vi "AD9959controlMR1_B2.vi"(9 "Enable Master Stepper":bool, 10 "Array":T2(array[cluster]) {"Sweep Parameters"."Rising Step Interval (ms)" min=0.0 max=2.55 step=0.01 format="%.2f"; "Sweep Parameters"."Stop Frequency (MHz)" min=0.0 max=400.0 step=1.0 format="%.6f"; "Sweep Parameters"."Start Frequency (MHz)" min=0.0 max=400.0 step=1.0 format="%.6f"; "Sweep Parameters"."Falling Step Interval (ms)" min=0.0 max=2.55 step=0.01 format="%.2f"; "Sweep Parameters"."Falling Step Size (MHz)" min=0.0 max=400.0 step=0.1 format="%.6f"; "Sweep Parameters"."Rising Step Size (MHz)" min=0.0 max=400.0 step=0.1 format="%.6f"; "ASF" min=0.0 max=1.0 step=0.001 format="%.3f"; "Channel Frequency (MHz)" min=0.0 max=400.0 step=1.0 format="%.6f"}, 11 "VISA Reference":refnum<visa-resource-name>="AD2") -> (2 "Duration array":T1(array[cluster]))   [LabVIEW 2016]
uses:
  <userlib>/configTool/configTool.llb/initConfigGlobal.vi
  <userlib>/configTool/configTool.llb/addProperty(DBL).vi
  <userlib>/configTool/configTool.llb/addProperty(BOOL).vi
  <userlib>/configTool/configTool.llb/saveConfigFile - Text.vi
  <userlib>/configTool/configTool.llb/closeConfig.vi
panel:
  out "Actual Channel Frequencies (MHz)":dbl[](array[numeric]) format="%#_10g"
  out "error out 2":errorcluster
  in  "config file path":path
  in  "Save Config File":bool=TRUE
  in  "Load Config File?":bool=TRUE
  out "System Clock (MHz)":u32
  in  "Multiplier":u32=5
  in  "Reference Clock (MHz)":u32=20
  # "AD2"
  # "AOM3    IntraAction 110 MHz\nRepump"
  # "AOM3    IntraAction 110MHz    \nWrite"
  # "AOM2   IntraAction 110 MHz\nRead"
  # "AOM7 Isomet 80MHz\nSPAD Gate"
  # "max 0.140"
  # "max 0.15"
  # "max 0.175"
  # "max 0.090/ 0.25 for LW"
  # "Channel 1"
  # "Channel 2"
  # "Channel 3"
  # "Channel 0"
  # "I/O"
  # "Clock"
  # "Profile Pins"
  # "P0 is uncut\nP1 is uncut\nP2 is uncut\nP3 is uncut"
  # "Power Down"
  # "Notes:\nMinimum Frequency Step is 0.0931 Hz.\nMinimum ASF Step is 0.001"
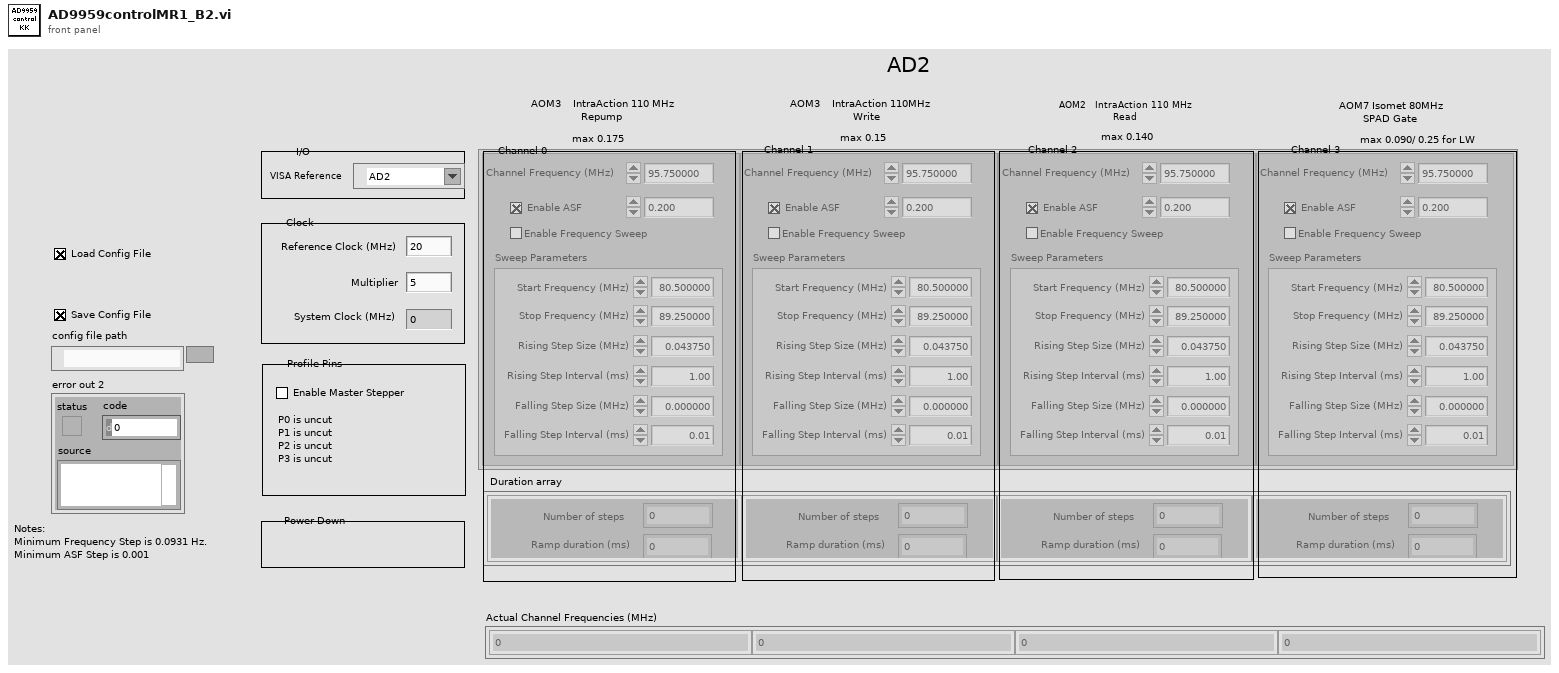
[diagram p1: front panel]
types:
  T1 = cluster{"Number of steps":dbl, "Ramp duration (ms)":dbl}[]
  T2 = cluster{"Enable ASF?":bool, "Channel Frequency (MHz)":dbl, "ASF":dbl, "Enable Frequency Sweep":bool, "Sweep Parameters":cluster{"Start Frequency (MHz)":dbl, "Stop Frequency (MHz)":dbl, "Rising Step Size (MHz)":dbl, "Falling Step Size (MHz)":dbl, "Falling Step Interval (ms)":dbl, "Rising Step Interval (ms)":dbl}}[]
  T3 = cluster{"Start Frequency (MHz)":dbl, "Stop Frequency (MHz)":dbl, "Rising Step Size (MHz)":dbl, "Falling Step Size (MHz)":dbl, "Falling Step Interval (ms)":dbl, "Rising Step Interval (ms)":dbl}[]
  T4 = cluster{"# of steps":dbl, "Ramp duration (ms)":dbl}[]
  T5 = cluster{"# of steps":dbl, "Ramp duration (ms)":dbl}
  T6 = cluster{"Start Frequency (MHz)":dbl, "Stop Frequency (MHz)":dbl, "Rising Step Size (MHz)":dbl, "Falling Step Size (MHz)":dbl, "Falling Step Interval (ms)":dbl, "Rising Step Interval (ms)":dbl}
  T7 = typedef "configRef.ctl" = refnum<vi>
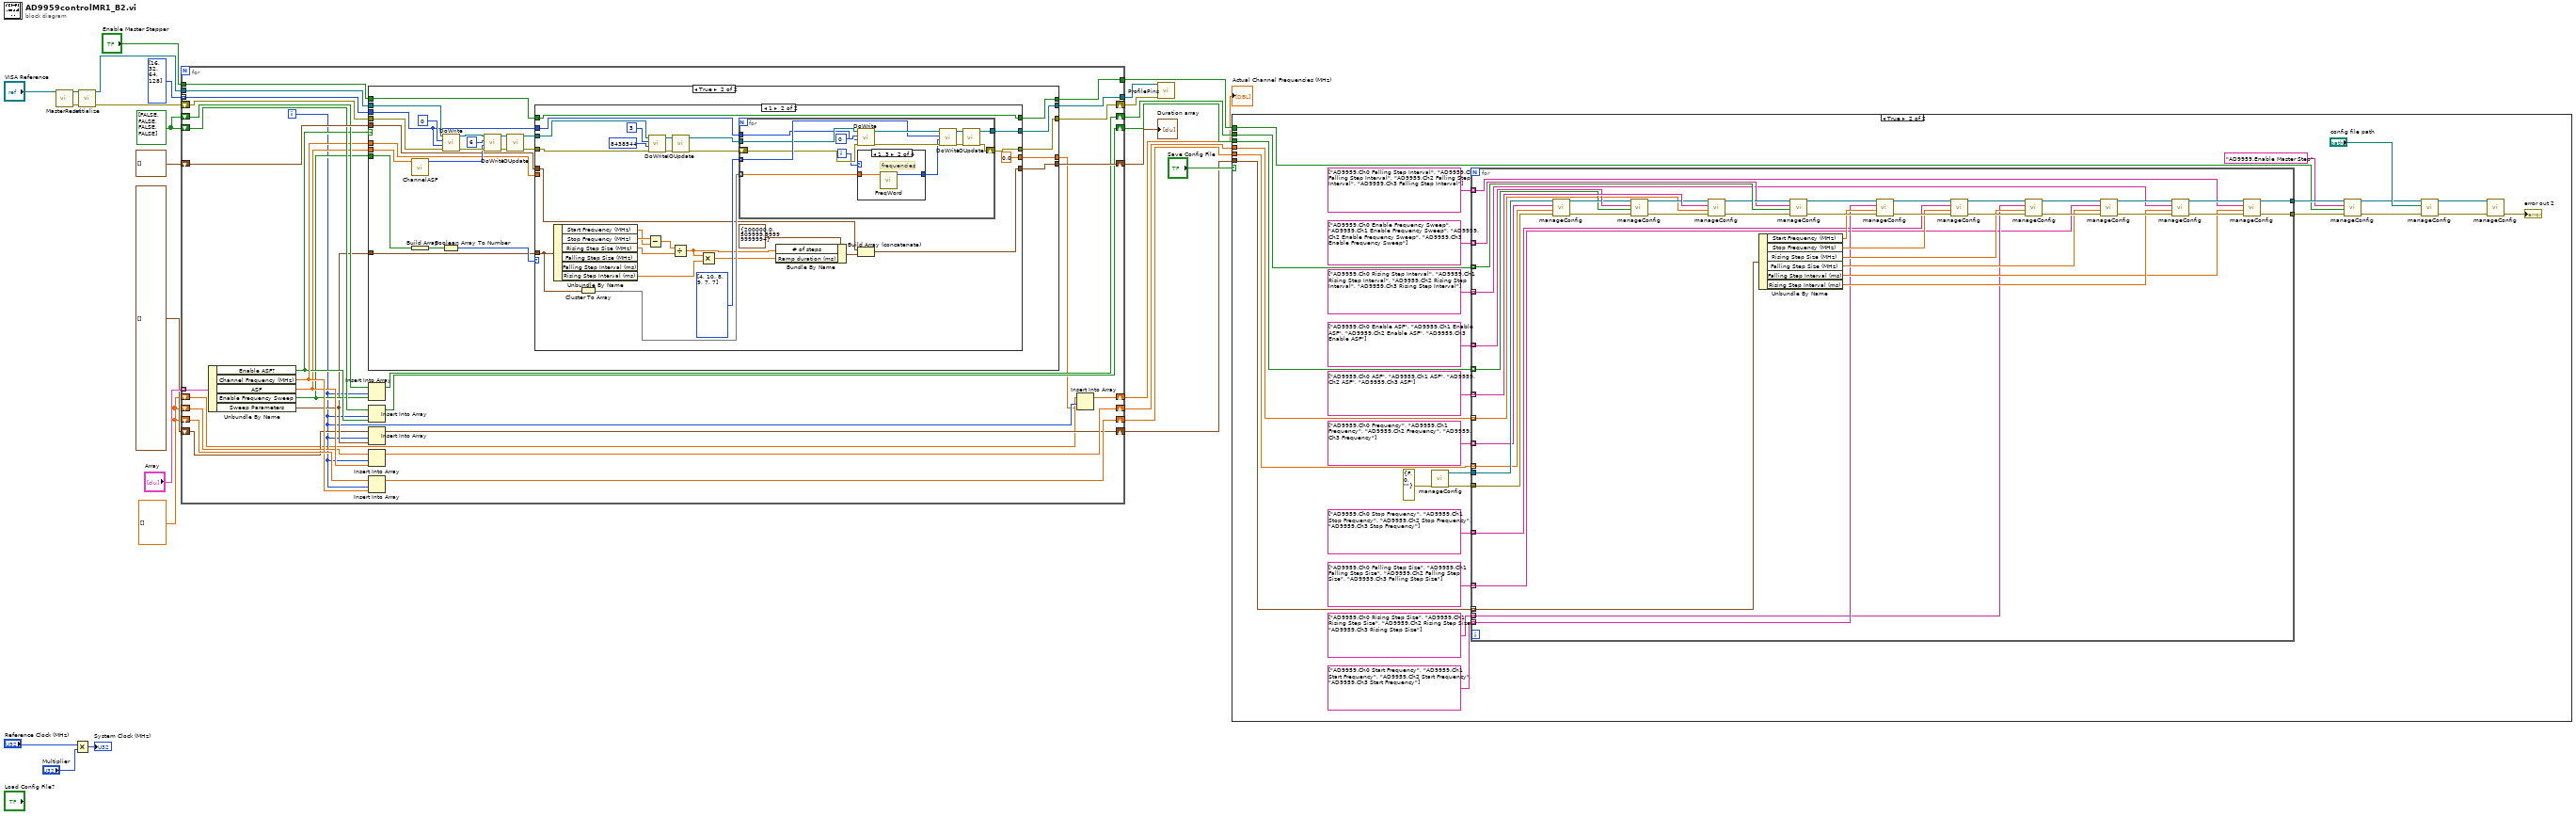
[diagram p0: block diagram]
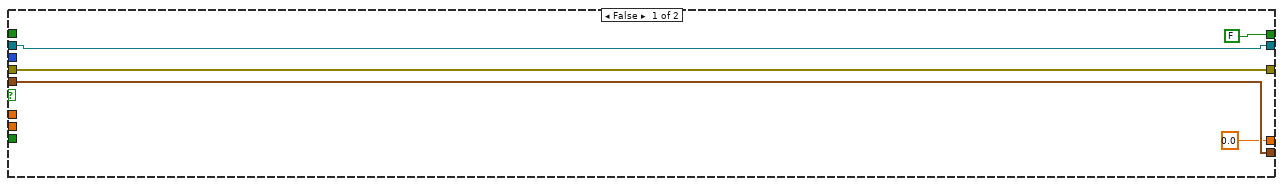
[diagram p3: hidden frame]
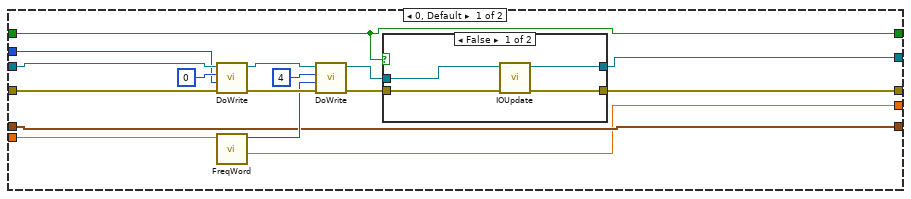
[diagram p4: hidden frame]
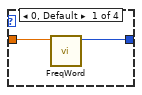
[diagram p6: hidden frame]
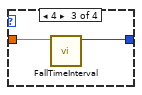
[diagram p7: hidden frame]
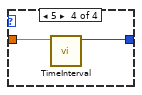
[diagram p8: hidden frame]
diagram:
  w2 = dbl[] [] ("array")
  w12 = bool[] [FALSE, FALSE, FALSE, FALSE] ("element")
  n1 = call "MasterReset.vi"("VISA Reference"="VISA Reference") -> ("error out"=w21:errorcluster, "dup VISA resource name"=w22:refnum<visa-resource-name>)  [unwired: 9 in]
  n2 = Multiply(x="Reference Clock (MHz)", y="Multiplier") -> (x*y=→"System Clock (MHz)":u32)
  n3 = call "Initialize.vi"("error in (no error)"=w21, "VISA Reference"=w22) -> ("error out"=w18:errorcluster, "dup VISA resource name"=w4:refnum<visa-resource-name>)  [unwired: 8 in]
  n4 = for {
    tunnel: "Array" -> [w55] mode=indexing
    tunnel: [w54] -> w3
    tunnel: w4 -> [w53]
    tunnel: u32[] [16, 32, 64, 128] ("Value 3") -> [w51] mode=indexing
    shift-right: [w50] -> w15
    shift-left: T4 [] -> [w49]
    shift-right: [w48] -> w19
    shift-left: w18 -> [w52]
    shift-right: [w46] -> w13
    shift-left: w12 -> [w47]
    shift-right: [w44] -> w11
    shift-left: w12 -> [w45]
    shift-right: [w41] -> w10
    shift-left: w2 -> [w43]
    shift-right: [w37] -> w8
    shift-left: w2 -> [w38]
    shift-right: [w33] -> w7
    shift-left: T3 [] ("array") -> [w34]
    tunnel: [w32] -> w6
    tunnel: "Enable Master Stepper" -> [w31]
    shift-right: [w28] -> w1
    shift-left: w2 -> [w29]
    i -> [w30]
    n5 = Unbundle By Name(w55) -> ("Enable ASF?"=w40:bool, "Channel Frequency (MHz)"=w42:dbl, "ASF"=w39:dbl, "Enable Frequency Sweep"=w36:bool, "Sweep Parameters"=w35:T6)
    n6 = case shown="True" w40 {
      tunnel: w53 -> [w60 w82]
      tunnel: w52 -> [w59 w83]
      tunnel: [w60 w74] -> w54
      tunnel: [w59 w73] -> w48
      tunnel: w39 -> [_ w72]
      tunnel: w36 -> [_ w67]
      tunnel: w42 -> [_ w71]
      tunnel: w35 -> [_ w62]
      tunnel: w51 -> [_ w70]
      tunnel: [w58 w66] -> w50
      tunnel: w49 -> [w58 w65]
      tunnel: [FALSE ("Enable Master Stepper") w64] -> w32
      tunnel: w31 -> [_ w63]
      tunnel: [0.0 ("Actual Frequency (MHz)") w61] -> w27
      frame False {
      }
      frame True {
        n7 = call "ChannelASF.vi"("ASF"=w72) -> ("ASF in hex"=w76:u32)  [unwired: 10 in]
        n8 = Build Array(w67) -> (w68:bool[])
        n9 = Boolean Array To Number(Boolean array=w68) -> (number=w69:u32)
        n10 = call "DoWrite.vi"("error in (no error)"=w83, "Value"=w70, "Register Address"=0 ("Value 3"), "VISA Reference"=w82) -> ("error out"=w79:errorcluster, "dup VISA resource name"=w81:refnum<visa-resource-name>)  [unwired: 6 in]
        n11 = call "DoWrite.vi"("error in (no error)"=w79, "Value"=w76, "Register Address"=u32 6 ("Register Address 4"), "VISA Reference"=w81) -> ("error out"=w77:errorcluster, "dup VISA resource name"=w80:refnum<visa-resource-name>)  [unwired: 6 in]
        n12 = call "IOUpdate.vi"("error in (no error)"=w77, "VISA Reference"=w80) -> ("error out"=w84:errorcluster, "dup VISA resource name"=w85:refnum<visa-resource-name>)  [unwired: 8 in]
        n13 = case shown="1" w69 {
          tunnel: w84 -> [w94 w131]
          tunnel: w85 -> [w101 w132]
          tunnel: [w92 w124] -> w74
          tunnel: [w91 w123] -> w73
          tunnel: w71 -> [w90 _]
          tunnel: w62 -> [_ w121]
          tunnel: w70 -> [w89 w122]
          tunnel: [w88 w110] -> w66
          tunnel: w65 -> [w88 w113]
          tunnel: [w87 w109] -> w64
          tunnel: w63 -> [w87 w109]
          tunnel: [w86 0.0 ("Actual Frequency (MHz)")] -> w61
          frame 0, Default {
            n14 = call "DoWrite.vi"("error in (no error)"=w94, "Value"=w89, "Register Address"=0 ("Value 3"), "VISA Reference"=w101) -> ("error out"=w100:errorcluster, "dup VISA resource name"=w99:refnum<visa-resource-name>)  [unwired: 6 in]
            n15 = call "FreqWord.vi"("Channel Frequency (MHz)"=w90) -> ("Actual Frequency (MHz)"=w86:dbl, "Frequency Tuning Word"=w95:u32)  [unwired: 9 in]
            n16 = call "DoWrite.vi"("error in (no error)"=w100, "Value"=w95, "Register Address"=u32 4 ("Register Address 2"), "VISA Reference"=w99) -> ("error out"=w97:errorcluster, "dup VISA resource name"=w98:refnum<visa-resource-name>)  [unwired: 6 in]
            n17 = case shown="False" w87 {
              tunnel: w98 -> [w105 w107]
              tunnel: w97 -> [w104 w106]
              tunnel: [w103 w107] -> w92
              tunnel: [w102 w106] -> w91
              frame False {
                n18 = call "IOUpdate.vi"("error in (no error)"=w104, "VISA Reference"=w105) -> ("error out"=w102:errorcluster, "dup VISA resource name"=w103:refnum<visa-resource-name>)  [unwired: 8 in]
              }
              frame True {
              }
            }
          }
          frame 1 {
            n19 = Unbundle By Name(w121) -> ("Start Frequency (MHz)"=w119:dbl, "Stop Frequency (MHz)"=w120:dbl, "Rising Step Size (MHz)"=w118:dbl, "Rising Step Interval (ms)"=w117:dbl)  [unwired: 2 out]
            n20 = Cluster To Array(cluster=w121) -> (array=w127:dbl[])
            n21 = Subtract(x=w120, y=w119) -> (x-y=w116:dbl)
            n22 = call "DoWrite.vi"("error in (no error)"=w131, "Value"=8438544 ("Value 3"), "Register Address"=3 ("Value 3"), "VISA Reference"=w132) -> ("error out"=w134:errorcluster, "dup VISA resource name"=w133:refnum<visa-resource-name>)  [unwired: 6 in]
            n23 = Divide(x=w116, y=w118) -> (x/y=w112:dbl)
            n24 = call "IOUpdate.vi"("error in (no error)"=w134, "VISA Reference"=w133) -> ("error out"=w126:errorcluster, "dup VISA resource name"=w125:refnum<visa-resource-name>)  [unwired: 8 in]
            n25 = Multiply(x=w112, y=w117) -> (x*y=w111:dbl)
            n26 = for {
              tunnel: i32[] [4, 10, 8, 9, 7, 7] -> [w144] mode=indexing
              shift-right: [w143] -> w123
              shift-left: w126 -> [w142]
              tunnel: w125 -> [w141]
              tunnel: [w136] -> w124
              tunnel: w127 -> [w138] mode=indexing
              tunnel: w122 -> [w135]
              i -> [w139]
              n27 = call "DoWrite.vi"("error in (no error)"=w142, "Value"=w135, "Register Address"=0 ("Value 3"), "VISA Reference"=w141) -> ("error out"=w145:errorcluster, "dup VISA resource name"=w146:refnum<visa-resource-name>)  [unwired: 6 in]
              n28 = case shown="1..3" w139 {
                tunnel: w138 -> [w150 w152 w154 w156]
                tunnel: [w149 w151 w153 w155] -> w137
                frame 0, Default {
                  n29 = call "FreqWord.vi"("Channel Frequency (MHz)"=w150) -> ("Frequency Tuning Word"=w149:u32)  [unwired: 9 in, 1 out]
                }
                frame 1..3 {
                  # "frequencies"
                  n30 = call "FreqWord.vi"("Channel Frequency (MHz)"=w152) -> ("Frequency Tuning Word"=w151:u32)  [unwired: 9 in, 1 out]
                }
                frame 4 {
                  n31 = call "FallTimeInterval.vi"("Fall Time Interval"=w154) -> ("Time interval in Hex"=w153:u32)  [unwired: 10 in]
                }
                frame 5 {
                  n32 = call "TimeInterval.vi"("Time Interval"=w156) -> ("Time interval in Hex"=w155:u32)  [unwired: 10 in]
                }
              }
              n33 = call "DoWrite.vi"("error in (no error)"=w145, "Value"=w137, "Register Address"=w144, "VISA Reference"=w146) -> ("error out"=w147:errorcluster, "dup VISA resource name"=w148:refnum<visa-resource-name>)  [unwired: 6 in]
              n34 = call "IOUpdate.vi"("error in (no error)"=w147, "VISA Reference"=w148) -> ("error out"=w143:errorcluster, "dup VISA resource name"=w136:refnum<visa-resource-name>)  [unwired: 8 in]
            }
            n35 = Bundle By Name(cluster=T5 {"# of steps"=200000.0, "Ramp duration (ms)"=509999.99999999994} ("Duration Cluster"), "# of steps"=w112, "Ramp duration (ms)"=w111) -> (w115:T5)
            n36 = Build Array (concatenate)(w113, w115) -> (w110:T4)
          }
        }
      }
    }
    n37 = Insert Into Array(array=w45, index=w30, new element=w36) -> (w44:bool[])
    n38 = Insert Into Array(array=w47, index=w30, new element=w40) -> (w46:bool[])
    n39 = Insert Into Array(array=w34, index=w30, new element=w35) -> (w33:T3)
    n40 = Insert Into Array(array=w38, index=w30, new element=w39) -> (w37:dbl[])
    n41 = Insert Into Array(array=w43, index=w30, new element=w42) -> (w41:dbl[])
    n42 = Insert Into Array(array=w29, index=w30, new element=w27) -> (w28:dbl[])
  }
  "Duration array" <- w15
  "Actual Channel Frequencies (MHz)" <- w1
  n43 = call "ProfilePins.vi"("error in (no error)"=w19, "VISA Reference"=w3) -> ()  [unwired: 8 in, 2 out]
  n44 = case shown="True" "Save Config File" {
    tunnel: w13 -> [_ w177]
    tunnel: w11 -> [_ w175]
    tunnel: w10 -> [_ w172]
    tunnel: w8 -> [_ w171]
    tunnel: w7 -> [_ w169]
    tunnel: w6 -> [_ w157]
    frame False {
    }
    frame True {
      n45 = call-poly <userlib>:"manageConfig.vi"("error in (no error)"=errorcluster {"status"=FALSE, "code"=0, "source"=""}) -> ("error out"=w174:errorcluster, "config ref out"=w179:T7)  [unwired: 9 in]
      n46 = for {
        tunnel: w179 -> [w222]
        tunnel: [w186] -> w162
        tunnel: string[] ["AD9959.Ch0 ASF", "AD9959.Ch1 ASF", "AD9959.Ch2 ASF", "AD9959.Ch3 ASF"] ("property path") -> [w227] mode=indexing
        tunnel: w177 -> [w217] mode=indexing
        tunnel: [w185] -> w161
        tunnel: string[] ["AD9959.Ch0 Enable ASF", "AD9959.Ch1 Enable ASF", "AD9959.Ch2 Enable ASF", "AD9959.Ch3 Enable ASF"] ("property path") -> [w225] mode=indexing
        tunnel: w175 -> [w214] mode=indexing
        tunnel: w174 -> [w220]
        tunnel: string[] ["AD9959.Ch0 Frequency", "AD9959.Ch1 Frequency", "AD9959.Ch2 Frequency", "AD9959.Ch3 Frequency"] ("property path") -> [w219] mode=indexing
        tunnel: w172 -> [w218] mode=indexing
        tunnel: w171 -> [w216] mode=indexing
        tunnel: string[] ["AD9959.Ch0 Enable Frequency Sweep", "AD9959.Ch1 Enable Frequency Sweep", "AD9959.Ch2 Enable Frequency Sweep", "AD9959.Ch3 Enable Frequency Sweep"] ("property path") -> [w212] mode=indexing
        tunnel: w169 -> [w211] mode=indexing
        tunnel: string[] ["AD9959.Ch0 Start Frequency", "AD9959.Ch1 Start Frequency", "AD9959.Ch2 Start Frequency", "AD9959.Ch3 Start Frequency"] ("property path") -> [w192] mode=indexing
        tunnel: string[] ["AD9959.Ch0 Stop Frequency", "AD9959.Ch1 Stop Frequency", "AD9959.Ch2 Stop Frequency", "AD9959.Ch3 Stop Frequency"] ("property path") -> [w191] mode=indexing
        tunnel: string[] ["AD9959.Ch0 Rising Step Size", "AD9959.Ch1 Rising Step Size", "AD9959.Ch2 Rising Step Size", "AD9959.Ch3 Rising Step Size"] ("property path") -> [w190] mode=indexing
        tunnel: string[] ["AD9959.Ch0 Falling Step Size", "AD9959.Ch1 Falling Step Size", "AD9959.Ch2 Falling Step Size", "AD9959.Ch3 Falling Step Size"] ("property path") -> [w189] mode=indexing
        tunnel: string[] ["AD9959.Ch0 Rising Step Interval", "AD9959.Ch1 Rising Step Interval", "AD9959.Ch2 Rising Step Interval", "AD9959.Ch3 Rising Step Interval"] ("property path") -> [w188] mode=indexing
        tunnel: string[] ["AD9959.Ch0 Falling Step Interval", "AD9959.Ch1 Falling Step Interval", "AD9959.Ch2 Falling Step Interval", "AD9959.Ch3 Falling Step Interval"] ("property path") -> [w187] mode=indexing
        n47 = call-poly <userlib>:"manageConfig.vi"("error in (no error)"=w220, "value"=w218, "property path"=w219, "config ref"=w222) -> ("error out"=w221:errorcluster, "config ref out"=w223:T7)  [unwired: 6 in]
        n48 = call-poly <userlib>:"manageConfig.vi"("error in (no error)"=w221, "value"=w217, "property path"=w225, "config ref"=w223) -> ("error out"=w224:errorcluster, "config ref out"=w226:T7)  [unwired: 6 in]
        n49 = call-poly <userlib>:"manageConfig.vi"("error in (no error)"=w224, "value"=w216, "property path"=w227, "config ref"=w226) -> ("error out"=w215:errorcluster, "config ref out"=w213:T7)  [unwired: 6 in]
        n50 = Unbundle By Name(w211) -> ("Start Frequency (MHz)"=w198:dbl, "Stop Frequency (MHz)"=w197:dbl, "Rising Step Size (MHz)"=w196:dbl, "Falling Step Size (MHz)"=w195:dbl, "Falling Step Interval (ms)"=w193:dbl, "Rising Step Interval (ms)"=w194:dbl)
        n51 = call-poly <userlib>:"manageConfig.vi"("error in (no error)"=w215, "value"=w214, "property path"=w212, "config ref"=w213) -> ("error out"=w199:errorcluster, "config ref out"=w200:T7)  [unwired: 6 in]
        n52 = call-poly <userlib>:"manageConfig.vi"("error in (no error)"=w199, "value"=w198, "property path"=w192, "config ref"=w200) -> ("error out"=w205:errorcluster, "config ref out"=w210:T7)  [unwired: 6 in]
        n53 = call-poly <userlib>:"manageConfig.vi"("error in (no error)"=w205, "value"=w197, "property path"=w191, "config ref"=w210) -> ("error out"=w204:errorcluster, "config ref out"=w209:T7)  [unwired: 6 in]
        n54 = call-poly <userlib>:"manageConfig.vi"("error in (no error)"=w204, "value"=w196, "property path"=w190, "config ref"=w209) -> ("error out"=w203:errorcluster, "config ref out"=w208:T7)  [unwired: 6 in]
        n55 = call-poly <userlib>:"manageConfig.vi"("error in (no error)"=w203, "value"=w195, "property path"=w189, "config ref"=w208) -> ("error out"=w202:errorcluster, "config ref out"=w207:T7)  [unwired: 6 in]
        n56 = call-poly <userlib>:"manageConfig.vi"("error in (no error)"=w202, "value"=w194, "property path"=w188, "config ref"=w207) -> ("error out"=w201:errorcluster, "config ref out"=w206:T7)  [unwired: 6 in]
        n57 = call-poly <userlib>:"manageConfig.vi"("error in (no error)"=w201, "value"=w193, "property path"=w187, "config ref"=w206) -> ("error out"=w185:errorcluster, "config ref out"=w186:T7)  [unwired: 6 in]
      }
      n58 = call-poly <userlib>:"manageConfig.vi"("error in (no error)"=w161, "value"=w157, "property path"="AD9959.Enable Master Step", "config ref"=w162) -> ("error out"=w160:errorcluster, "config ref out"=w159:T7)  [unwired: 6 in]
      n59 = call-poly <userlib>:"manageConfig.vi"("error in"=w160, "config file path"="config file path", "config ref"=w159) -> ("error out"=w184:errorcluster, "config ref out"=w183:T7)  [unwired: 6 in, 1 out]
      n60 = call-poly <userlib>:"manageConfig.vi"("error in (no error)"=w184, "config ref"=w183) -> ("error out"=→"error out 2":errorcluster)  [unwired: 9 in]
    }
  }
